vi "Repo Page Finder.vi"() -> ()   [LabVIEW 2023]
uses:
  Repo Page Finder Action.ctl
  <vilib>/Wiresmith Technology/G CLI/CLI Class/CLI.lvclass
  Confluence Settings.ctl
  <vilib>/Wiresmith Technology/G CLI/Argument Parser/Option Class/Option Configuration.ctl
  <vilib>/Wiresmith Technology/G CLI/Argument Parser/Option Class/Argument Type.ctl
  <userlib>/_PetranWay/LabVIEW Confluence API/Source/Confluence/Page/Page.lvclass/Page.ctl
  <vilib>/Wiresmith Technology/G CLI/CLI Class/Output.ctl
  fd638966-1e81-4a6e-910d-8f77ad7d0e1b.vi
  <userlib>/_PetranWay/LabVIEW Confluence API/Source/Confluence/Page/Accessors/Read title.vi
  <userlib>/_PetranWay/LabVIEW Confluence API/Source/Confluence/Page/Accessors/Read ID.vi
  <vilib>/JDP Science/JSONtext/Find Item.vi
  <userlib>/_PetranWay/LabVIEW Atlassian API/Source/JSON Utilities/Strip Quotes Around String.vi
  <vilib>/JDP Science/JSONtext/Next JSON Value.vi
  <vilib>/JDP Science/JSONtext/String Subset.vi
  <vilib>/JDP Science/JSONtext/Parsing/Advance past next JSON Value (inlined COPY).vi
  <vilib>/JDP Science/JSONtext/Parsing/Advance past whitespace.vi
  <vilib>/JDP Science/JSONtext/Parsing/Advance past String.vi
  <vilib>/JDP Science/JSONtext/Parsing/Advance past Number.vi
  <vilib>/JDP Science/JSONtext/Parsing/Advance past Line Ending.vi
  <vilib>/JDP Science/JSONtext/Parsing/Parse Full Path or Item Name.vi
  <vilib>/JDP Science/JSONtext/Parsing/Advance past Array.vi
  <vilib>/JDP Science/JSONtext/Parsing/Advance past Object.vi
  <vilib>/JDP Science/JSONtext/support/Error Cluster From Code.vi
  <vilib>/JDP Science/JSONtext/Offset/Find Item Locations by Path.vi
  <userlib>/_PetranWay/LabVIEW Confluence API/Source/Confluence/Confluence Connection/Confluence.lvclass
  <userlib>/_PetranWay/LabVIEW Confluence API/Source/Confluence/iConfluence/iConfluence.lvclass
  <userlib>/_PetranWay/LabVIEW Confluence API/Source/Confluence/Page/Page.lvclass
  <vilib>/Wiresmith Technology/G CLI/Argument Parser/Option Class/Option.lvclass
  <vilib>/Wiresmith Technology/G CLI/Argument Parser/Option Set Class/Option Set.lvclass
panel:
  out "Scoped Access Token?":bool
  out "Repo Name":string
  out "Custom Parameters":string[](array[string])
  out "Confluence Token":string
  out "Confluence Email":string
  out "Confluence URL":string
  out "Use Data Center for Confluence Connection?":bool
  out "Use Login INI file for Confluence Connection?":bool
  out "Top Page ID":string
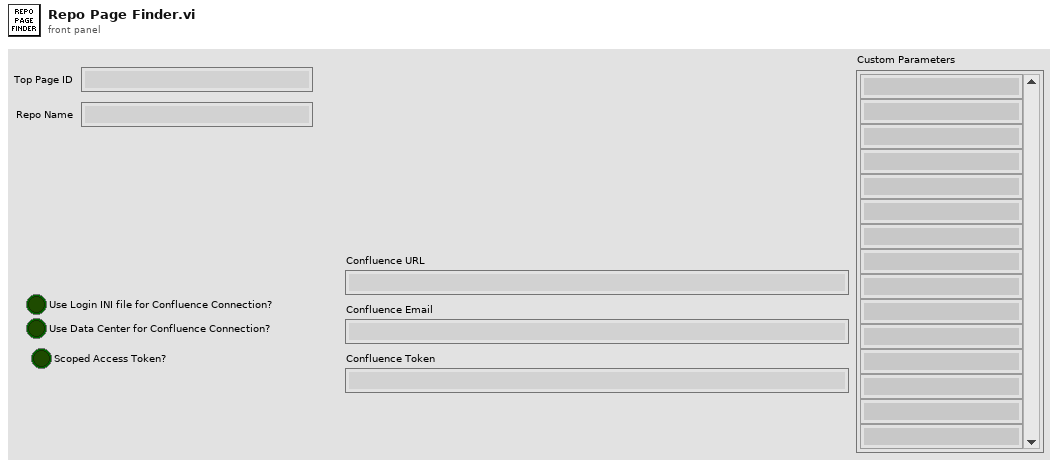
[diagram p1: front panel]
types:
  T1 = typedef "Confluence Settings.ctl" = cluster{"Use INI?":bool, "URL":string, "Email":string, "Token":string, "Use Settings File?":bool, "Data Center?":bool, "Scoped Token?":bool}
  T2 = cluster{"CLI":refnum<class "CLI.lvclass">, "Working Directory":path, "Top Page ID":string, "Confluence Settings":T1, "Repo Name":string, "Repo Page ID":string}
  T3 = typedef "Repo Page Finder Action.ctl" = enum16{"Initialize", "Find Repo Page", "Close", "Help"}
  T4 = enum16{"Top Page ID", "Repo Name", "Confluence Use INI", "Confluence Type", "Confluence URL", "Confluence Email", "Confluence Token", "Scoped Token"}
  T5 = typedef "Option Parser.lvlib/Option.lvclass/Option Configuration.ctl" = cluster{"Option Type":T6, "Option Labels":string[], "Key":string, "Description":string, "Required":bool, "Default Value":string}
  T6 = typedef "Option Parser.lvlib/Option.lvclass/Argument Type.ctl" = enum16{"flag", "value"}
  T7 = typedef "CLI.lvclass/Output.ctl" = enum16{"StdOut", "StdErr"}
  T8 = enum16{"Top Page ID", "Repo Name", "Confluence Use INI", "Confluence Type", "Confluence URL", "Confluence Email", "Confluence Token", "Scoped Token"}[]
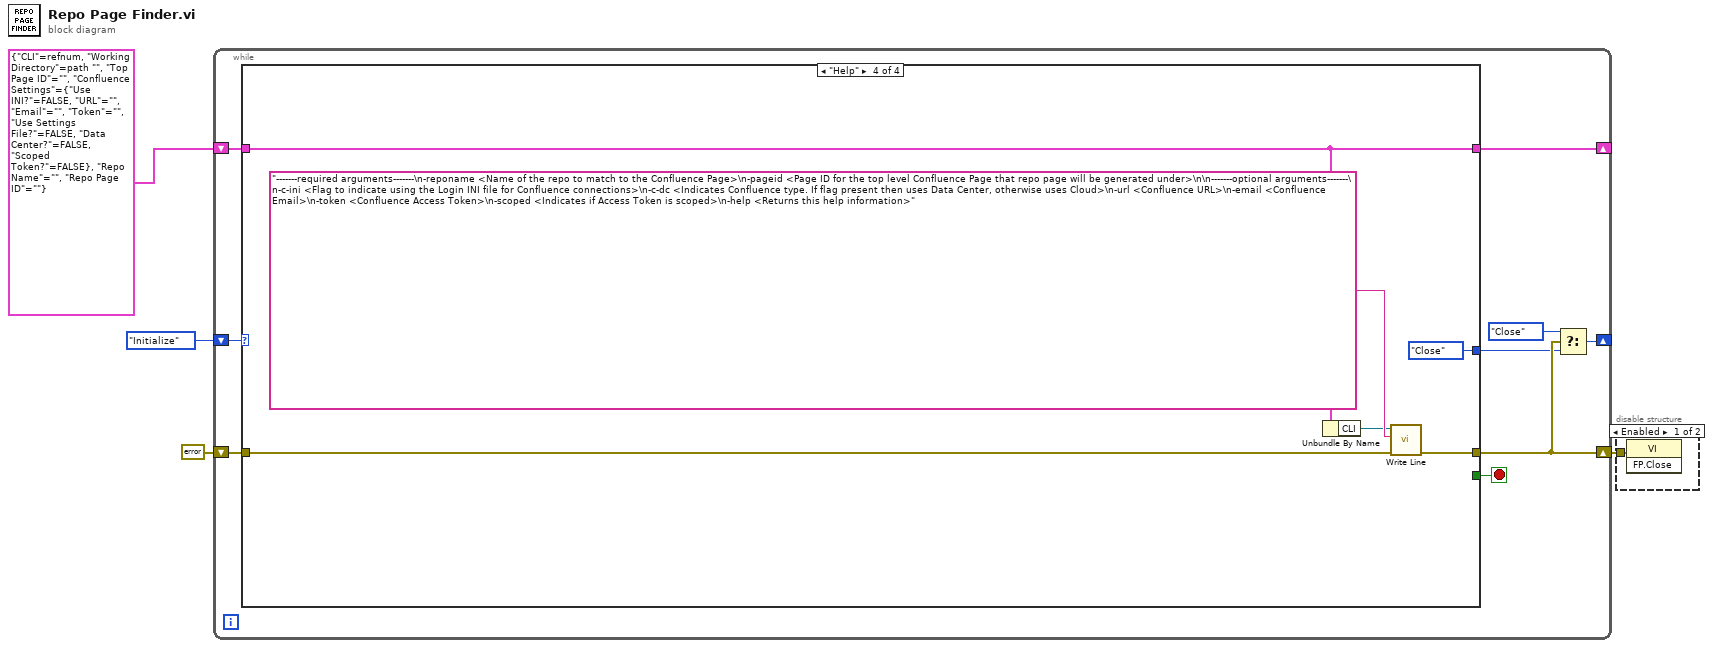
[diagram p0: block diagram]
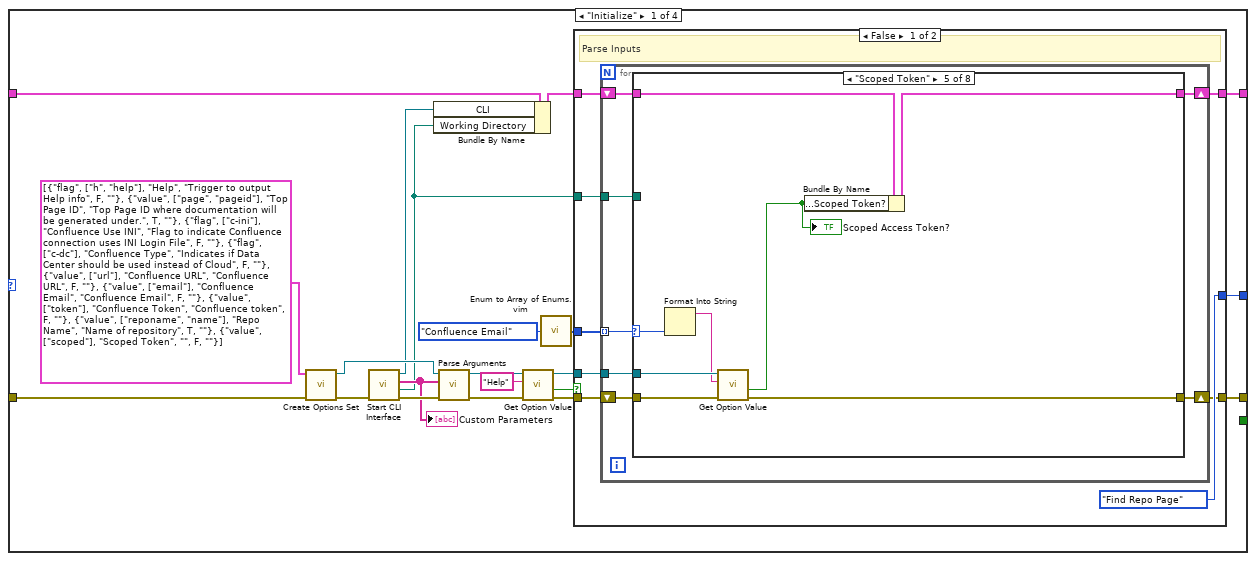
[diagram p3: hidden frame]
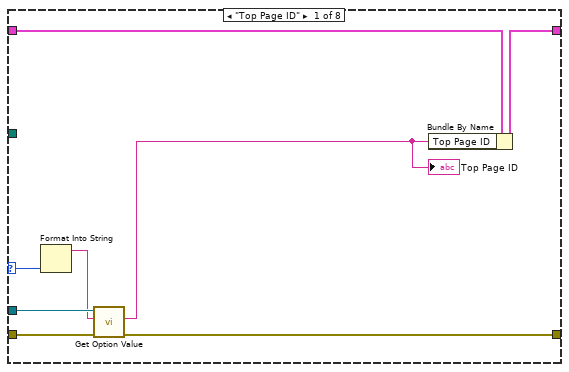
[diagram p4: hidden frame]
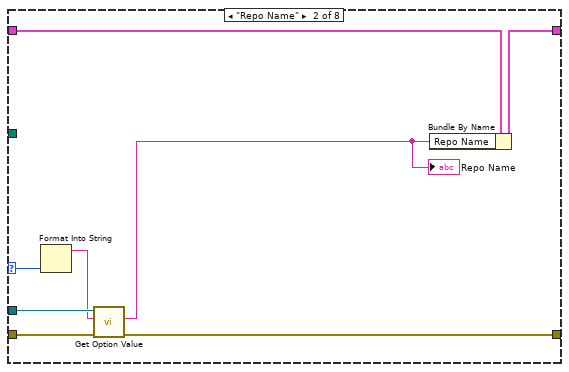
[diagram p5: hidden frame]
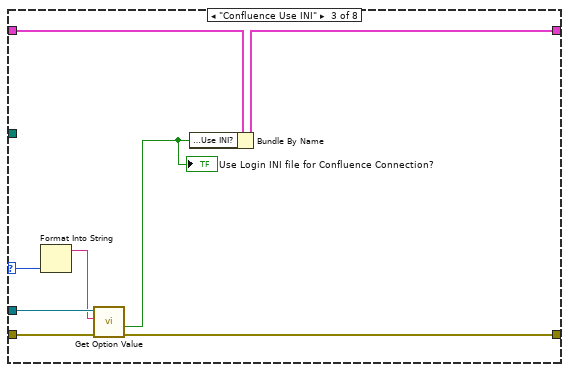
[diagram p6: hidden frame]
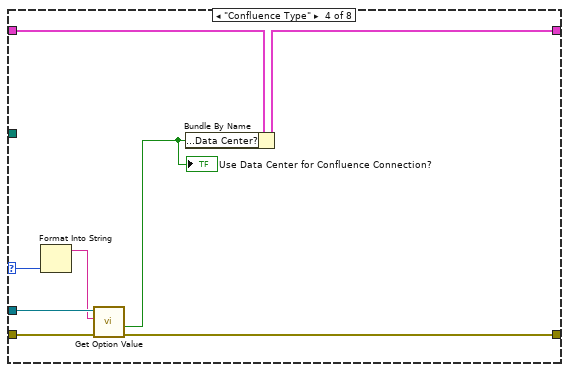
[diagram p7: hidden frame]
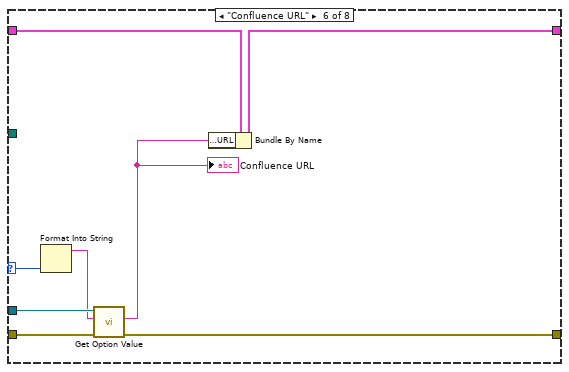
[diagram p8: hidden frame]
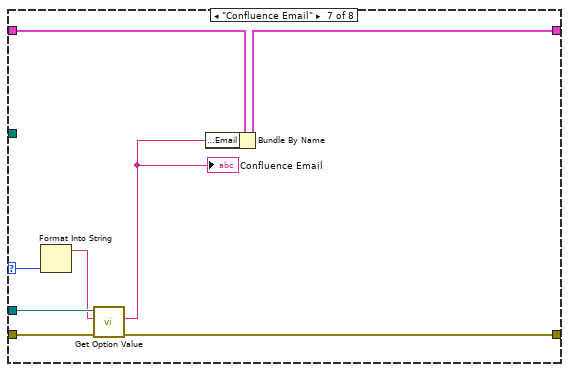
[diagram p9: hidden frame]
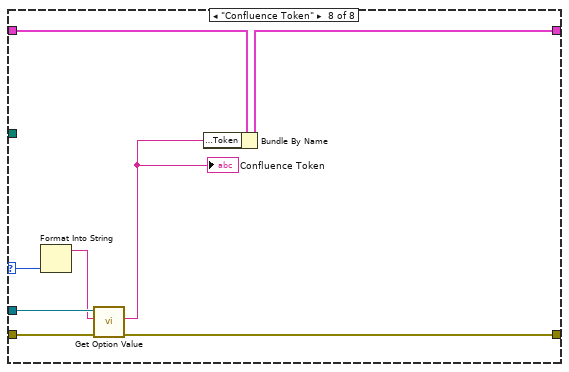
[diagram p10: hidden frame]
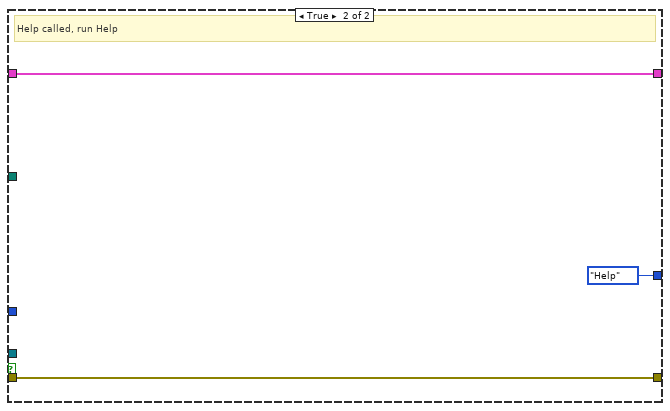
[diagram p11: hidden frame]
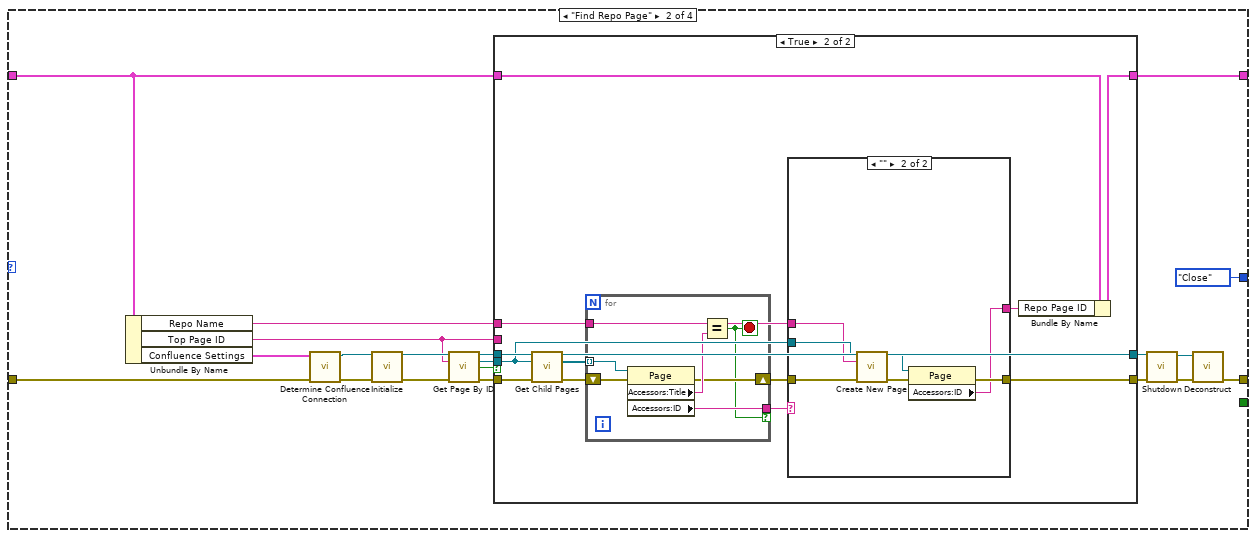
[diagram p12: hidden frame]
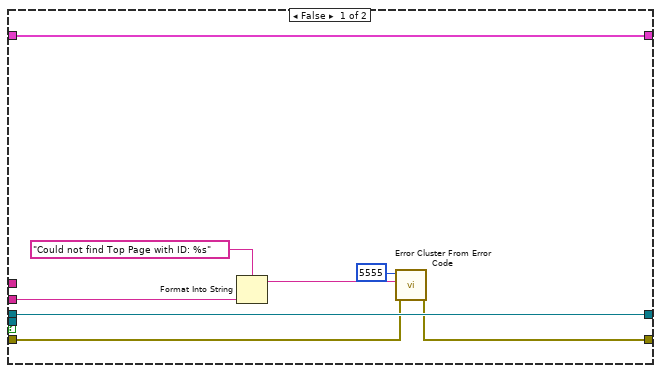
[diagram p13: hidden frame]
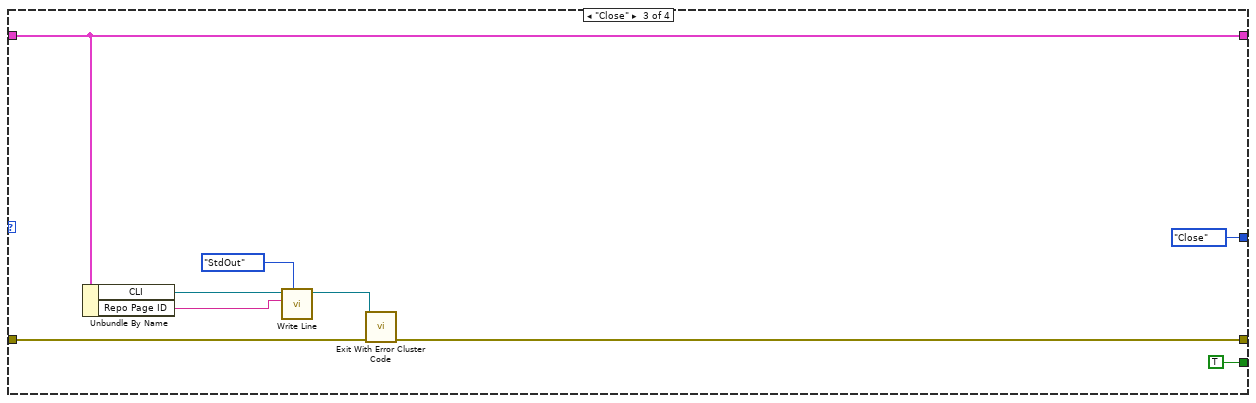
[diagram p15: hidden frame]
diagram:
  n1 = while {
    shift-right: [w8] -> _
    shift-left: Repo_Page_Finder_Action."Initialize" -> [w13]
    shift-right: [w10] -> w2
    shift-left: errorcluster {"status"=FALSE, "code"=0, "source"=""} ("error out") -> [w12]
    shift-right: [w5] -> _
    shift-left: T2 {"CLI"=refnum, "Working Directory"=path "", "Top Page ID"="", "Confluence Settings"={"Use INI?"=FALSE, "URL"="", "Email"="", "Token"="", "Use Settings File?"=FALSE, "Data Center?"=FALSE, "Scoped Token?"=FALSE}, "Repo Name"="", "Repo Page ID"=""} -> [w6]
    stop <- w7 stop-if-true
    n2 = case shown="\"Help\"" w13 {
      tunnel: w12 -> [w26 w134 w177 w186]
      tunnel: [w17 w122 w178 w187] -> w10
      tunnel: [w19 Repo_Page_Finder_Action."Close" Repo_Page_Finder_Action."Close" Repo_Page_Finder_Action."Close"] -> w9
      tunnel: [_ _ TRUE _] -> w7
      tunnel: w6 -> [w25 w117 w180 w184]
      tunnel: [w21 w118 w180 w184] -> w5
      frame "Initialize" {
        n3 = call <vilib>:"Create Options Set.vi"("error in (no error)"=w26, "Options"=T5[] [{"Option Type"=enum."flag", "Option Labels"=["h", "help"], "Key"="Help", "Description"="Trigger to output Help info", "Required"=FALSE, "Default Value"=""}, {"Option Type"=enum."value", "Option Labels"=["page", "pageid"], "Key"="Top Page ID", "Description"="Top Page ID where documentation will be generated under.", "Required"=TRUE, "Default Value"=""}, {"Option Type"=enum."flag", "Option Labels"=["c-ini"], "Key"="Confluence Use INI", "Description"="Flag to indicate Confluence connection uses INI Login File", "Required"=FALSE, "Default Value"=""}, {"Option Type"=enum."flag", "Option Labels"=["c-dc"], "Key"="Confluence Type", "Description"="Indicates if Data Center should be used instead of Cloud", "Required"=FALSE, "Default Value"=""}, {"Option Type"=enum."value", "Option Labels"=["url"], "Key"="Confluence URL", "Description"="Confluence URL", "Required"=FALSE, "Default Value"=""}, {"Option Type"=enum."value", "Option Labels"=["email"], "Key"="Confluence Email", "Description"="Confluence Email", "Required"=FALSE, "Default Value"=""}, {"Option Type"=enum."value", "Option Labels"=["token"], "Key"="Confluence Token", "Description"="Confluence token", "Required"=FALSE, "Default Value"=""}, {"Option Type"=enum."value", "Option Labels"=["reponame", "name"], "Key"="Repo Name", "Description"="Name of repository", "Required"=TRUE, "Default Value"=""}, {"Option Type"=enum."value", "Option Labels"=["scoped"], "Key"="Scoped Token", "Description"="", "Required"=FALSE, "Default Value"=""}]) -> ("error out"=w32:errorcluster, "Option Set out"=w31:refnum<class "Option Set.lvclass">)  [unwired: 8 in]
        n4 = call <vilib>:"Start CLI Interface.vi"("error in (no error)"=w32) -> ("error out"=w34:errorcluster, "Working Directory"=w14:path, "Custom Parameters"=w30:string[], "CLI out"=w24:refnum<class "CLI.lvclass">)  [unwired: 7 in]
        "Custom Parameters" <- w30
        n5 = Bundle By Name(cluster=w25, "CLI"=w24, "Working Directory"=w14) -> (w20:T2)
        n6 = call <vilib>:"Parse Arguments.vi"("error in (no error)"=w34, "Arguments"=w30, "Option Set in"=w31) -> ("error out"=w28:errorcluster, "Option Set out"=w27:refnum<class "Option Set.lvclass">)  [unwired: 5 in, 2 out]
        n7 = call <vilib>:"Get Option Value.vi"("error in (no error)"=w28, "Option Key"="Help", "Option Set in"=w27) -> ("error out"=w18:errorcluster, "Set"=w23:bool, "Option Set out"=w22:refnum<class "Option Set.lvclass">)  [unwired: 5 in, 1 out]
        n8 = call "Enum to Array of Enums.vim"("enum"=T4."Confluence Email") -> ("array of enums"=w15:T8)
        n9 = case shown="False" w23 {
          tunnel: w22 -> [w41 _]
          tunnel: [w39 w116] -> w21
          tunnel: w20 -> [w40 w116]
          tunnel: [Repo_Page_Finder_Action."Find Repo Page" Repo_Page_Finder_Action."Help"] -> w19
          tunnel: w18 -> [w42 w114]
          tunnel: [w35 w114] -> w17
          tunnel: w15 -> [w38 _]
          tunnel: w14 -> [w37 _]
          frame False {
            # "Parse Inputs"
            n10 = for {
              shift-right: [w44] -> w35
              shift-left: w42 -> [w45]
              tunnel: w41 -> [w46]
              shift-right: [w47] -> w39
              shift-left: w40 -> [w48]
              tunnel: w38 -> [w49] mode=indexing
              tunnel: w37 -> [w43]
              n11 = case shown="\"Scoped Token\"" w49 {
                selector: w49 -> [w54 w62 w70 w78 w86 w94 w102 w110]
                tunnel: w48 -> [w57 w65 w73 w81 w89 w97 w105 w113]
                tunnel: [w51 w59 w67 w75 w83 w91 w99 w107] -> w47
                tunnel: w46 -> [w55 w63 w71 w79 w87 w95 w103 w111]
                tunnel: w45 -> [w56 w64 w72 w80 w88 w96 w104 w112]
                tunnel: [w52 w60 w68 w76 w84 w92 w100 w108] -> w44
                tunnel: w43 -> [_ _ _ _ _ _ _ _]
                frame "Top Page ID" {
                  n12 = Format Into String(w54) -> (resulting string=w53:string)  [unwired: 3 in, 1 out]
                  n13 = call <vilib>:"Get Option Value.vi"("error in (no error)"=w56, "Option Key"=w53, "Option Set in"=w55) -> ("error out"=w52:errorcluster, "Value"=w50:string)  [unwired: 5 in, 2 out]
                  "Top Page ID" <- w50
                  n14 = Bundle By Name(cluster=w57, "Top Page ID"=w50) -> (w51:T2)
                }
                frame "Repo Name" {
                  n15 = Format Into String(w62) -> (resulting string=w61:string)  [unwired: 3 in, 1 out]
                  n16 = call <vilib>:"Get Option Value.vi"("error in (no error)"=w64, "Option Key"=w61, "Option Set in"=w63) -> ("error out"=w60:errorcluster, "Value"=w58:string)  [unwired: 5 in, 2 out]
                  "Repo Name" <- w58
                  n17 = Bundle By Name(cluster=w65, "Repo Name"=w58) -> (w59:T2)
                }
                frame "Confluence Use INI" {
                  n18 = Format Into String(w70) -> (resulting string=w69:string)  [unwired: 3 in, 1 out]
                  n19 = call <vilib>:"Get Option Value.vi"("error in (no error)"=w72, "Option Key"=w69, "Option Set in"=w71) -> ("error out"=w68:errorcluster, "Set"=w66:bool)  [unwired: 5 in, 2 out]
                  "Use Login INI file for Confluence Connection?" <- w66
                  n20 = Bundle By Name(cluster=w73, "Confluence Settings.Use INI?"=w66) -> (w67:T2)
                }
                frame "Confluence Type" {
                  n21 = Format Into String(w78) -> (resulting string=w77:string)  [unwired: 3 in, 1 out]
                  n22 = call <vilib>:"Get Option Value.vi"("error in (no error)"=w80, "Option Key"=w77, "Option Set in"=w79) -> ("error out"=w76:errorcluster, "Set"=w74:bool)  [unwired: 5 in, 2 out]
                  "Use Data Center for Confluence Connection?" <- w74
                  n23 = Bundle By Name(cluster=w81, "Confluence Settings.Data Center?"=w74) -> (w75:T2)
                }
                frame "Scoped Token" {
                  n24 = Format Into String(w86) -> (resulting string=w85:string)  [unwired: 3 in, 1 out]
                  n25 = call <vilib>:"Get Option Value.vi"("error in (no error)"=w88, "Option Key"=w85, "Option Set in"=w87) -> ("error out"=w84:errorcluster, "Set"=w82:bool)  [unwired: 5 in, 2 out]
                  "Scoped Access Token?" <- w82
                  n26 = Bundle By Name(cluster=w89, "Confluence Settings.Scoped Token?"=w82) -> (w83:T2)
                }
                frame "Confluence URL" {
                  n27 = Format Into String(w94) -> (resulting string=w93:string)  [unwired: 3 in, 1 out]
                  n28 = call <vilib>:"Get Option Value.vi"("error in (no error)"=w96, "Option Key"=w93, "Option Set in"=w95) -> ("error out"=w92:errorcluster, "Value"=w90:string)  [unwired: 5 in, 2 out]
                  "Confluence URL" <- w90
                  n29 = Bundle By Name(cluster=w97, "Confluence Settings.URL"=w90) -> (w91:T2)
                }
                frame "Confluence Email" {
                  n30 = Format Into String(w102) -> (resulting string=w101:string)  [unwired: 3 in, 1 out]
                  n31 = call <vilib>:"Get Option Value.vi"("error in (no error)"=w104, "Option Key"=w101, "Option Set in"=w103) -> ("error out"=w100:errorcluster, "Value"=w98:string)  [unwired: 5 in, 2 out]
                  "Confluence Email" <- w98
                  n32 = Bundle By Name(cluster=w105, "Confluence Settings.Email"=w98) -> (w99:T2)
                }
                frame "Confluence Token" {
                  n33 = Format Into String(w110) -> (resulting string=w109:string)  [unwired: 3 in, 1 out]
                  n34 = call <vilib>:"Get Option Value.vi"("error in (no error)"=w112, "Option Key"=w109, "Option Set in"=w111) -> ("error out"=w108:errorcluster, "Value"=w106:string)  [unwired: 5 in, 2 out]
                  "Confluence Token" <- w106
                  n35 = Bundle By Name(cluster=w113, "Confluence Settings.Token"=w106) -> (w107:T2)
                }
              }
            }
          }
          frame True {
            # "Help called, run Help"
          }
        }
      }
      frame "Find Repo Page" {
        n36 = Unbundle By Name(w117) -> ("Repo Name"=w119:string, "Top Page ID"=w120:string, "Confluence Settings"=w135:T1)
        n37 = call "Determine Confluence Connection.vi"("Error in"=w134, "Confluence Settings"=w135) -> ("Error out"=w133:errorcluster, "Confluence"=w132:refnum<class "Confluence.lvclass">)  [unwired: 8 in]
        n38 = call-dynamic "Initialize.vi"("Confluence in"=w132, "error in (no error)"=w133) -> ("Confluence out"=w131:refnum<class "Confluence.lvclass">, "error out"=w130:errorcluster)  [unwired: 12 in]
        n39 = call-dynamic "Get Page By ID.vi"("Confluence Connection in"=w131, "ID"=w120, "error in (no error)"=w130) -> ("Atlassian Connection out"=w129:refnum<class "Confluence.lvclass">, "Page out"=w127:refnum<class "Page.lvclass">, "Found"=w126:bool, "error out"=w128:errorcluster)  [unwired: 9 in]
        n40 = case shown="True" w126 {
          tunnel: w129 -> [w144 w157]
          tunnel: w128 -> [w142 w156]
          tunnel: w127 -> [_ w147]
          tunnel: [w143 w150] -> w125
          tunnel: [w144 w145] -> w121
          tunnel: w120 -> [w139 _]
          tunnel: w119 -> [_ w146]
          tunnel: [w137 w152] -> w118
          tunnel: w117 -> [w137 w153]
          frame False {
            n41 = Format Into String(format string="Could not find Top Page with ID: %s", w139) -> (resulting string=w138:string)  [unwired: 2 in, 1 out]
            n42 = call <vilib>:"Error Cluster From Error Code.vi"("error in (no error)"=w142, "error message (\"\")"=w138, "error code (0)"=5555) -> ("error out"=w143:errorcluster)  [unwired: 6 in]
          }
          frame True {
            n43 = call-dynamic "Get Child Pages.vi"("Confluence Connection in"=w157, "Page"=w147, "error in (no error)"=w156) -> ("Confluence Connection out"=w145:refnum<class "Confluence.lvclass">, "Child Pages"=w154:refnum<class "Page.lvclass">[], "error out"=w155:errorcluster)  [unwired: 9 in, 1 out]
            n44 = for {
              shift-right: [w169] -> w151
              shift-left: w155 -> [w172]
              tunnel: w154 -> [w173] mode=indexing
              tunnel: w146 -> [w171]
              tunnel: [w168] -> w149 if=w167
              stop <- w167 stop-if-true
              n45 = property class="Page"(reference=w173, error in=w172) -> (error out=w169:errorcluster, "Accessors:Title"=w170:string, "Accessors:ID"=w168:string)  [unwired: 1 out]
              n46 = Equal?(x=w171, y=w170) -> (x = y?=w167:bool)
            }
            n47 = case shown="\"\"" w149 {
              selector: w149 -> [w158 _]
              tunnel: w151 -> [w159 w166]
              tunnel: [w159 w162] -> w150
              tunnel: [w158 w160] -> w148
              tunnel: w147 -> [_ w165]
              tunnel: w146 -> [_ w164]
              frame Default {
                # "Page Already Exists"
              }
              frame "" {
                n48 = call-dynamic "Create New Page.vi"("Desired Parent Page"=w165, "New Page Title"=w164, "error in (no error)"=w166) -> ("Created Page"=w161:refnum<class "Page.lvclass">, "error out"=w163:errorcluster)  [unwired: 11 in]
                n49 = property class="Page"(reference=w161, error in=w163) -> (error out=w162:errorcluster, "Accessors:ID"=w160:string)  [unwired: 1 out]
              }
            }
            n50 = Bundle By Name(cluster=w153, "Repo Page ID"=w148) -> (w152:T2)
          }
        }
        n51 = call-dynamic "Shutdown.vi"("Confluence in"=w121, "error in (no error)"=w125) -> ("Confluence out"=w123:refnum<class "Confluence.lvclass">, "error out"=w124:errorcluster)  [unwired: 12 in]
        n52 = call-dynamic "Deconstruct.vi"("error in (no error)"=w124, "Confluence in"=w123) -> ("error out"=w122:errorcluster)  [unwired: 9 in]
      }
      frame "Close" {
        n53 = Unbundle By Name(w180) -> ("CLI"=w179:refnum<class "CLI.lvclass">, "Repo Page ID"=w174:string)
        n54 = call <vilib>:"Write Line.vi"("Output (StdOut)"=Output."StdOut", "Text to Write"=w174, "CLI in"=w179) -> ("CLI out"=w176:refnum<class "CLI.lvclass">)  [unwired: 7 in, 1 out]
        n55 = call <vilib>:"Exit With Error Cluster Code.vi"("error in (no error)"=w177, "CLI in"=w176) -> ("error out"=w178:errorcluster)  [unwired: 9 in]
      }
      frame "Help" {
        n56 = Unbundle By Name(w184) -> ("CLI"=w183:refnum<class "CLI.lvclass">)
        n57 = call <vilib>:"Write Line.vi"("error in (no error)"=w186, "Text to Write"="-------required arguments-------\n-reponame <Name of the repo to match to the Confluence Page>\n-pageid <Page ID for the top level Confluence Page that repo page will be generated under>\n\n-------optional arguments-------\n-c-ini <Flag to indicate using the Login INI file for Confluence connections>\n-c-dc <Indicates Confluence type. If flag present then uses Data Center, otherwise uses Cloud>\n-url <Confluence URL>\n-email <Confluence Email>\n-token <Confluence Access Token>\n-scoped <Indicates if Access Token is scoped>\n-help <Returns this help information>" ("string"), "CLI in"=w183) -> ("error out"=w187:errorcluster)  [unwired: 7 in, 1 out]
      }
    }
    n58 = Select(t=Repo_Page_Finder_Action."Close", s=w10, f=w9) -> (s? t:f=w8:T3)
  }
  n59 = disable-structure shown="Enabled" {
    disable-tunnel: w2 -> [w189 _]
    frame Enabled {
      n60 = invoke class="VI" method="FP.Close"(error in=w189) -> ()  [unwired: 2 in, 3 out]
    }
    frame Disabled {
    }
  }
